vi "Excercise 2.vi"() -> ()   [LabVIEW 2017]
panel:
  in  "Score 3":dbl
  in  "Score 2":dbl
  out "Numeric 1":dbl
  in  "Score 1":dbl
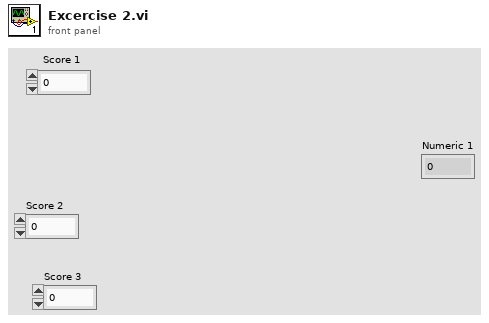
[diagram p1: front panel]
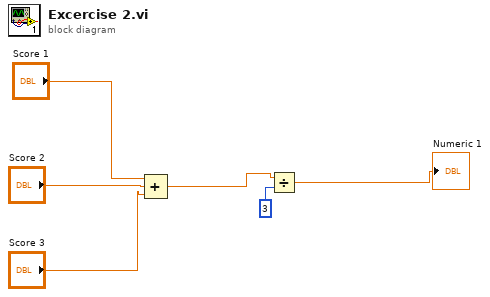
[diagram p0: block diagram]
diagram:
  n1 = Compound Arithmetic op=ADD("Score 1", "Score 2", "Score 3") -> (w2:dbl)
  n2 = Divide(x=w2, y=3) -> (x/y=→"Numeric 1":dbl)
